vi "SelectWindow(SubVI).vi"(11 "Permanent data":T1) -> (0 "Error Out":errorcluster, 3 "Manometr out":T1)   [LabVIEW 2018]
uses:
  PressureGaugeInfo.ctl
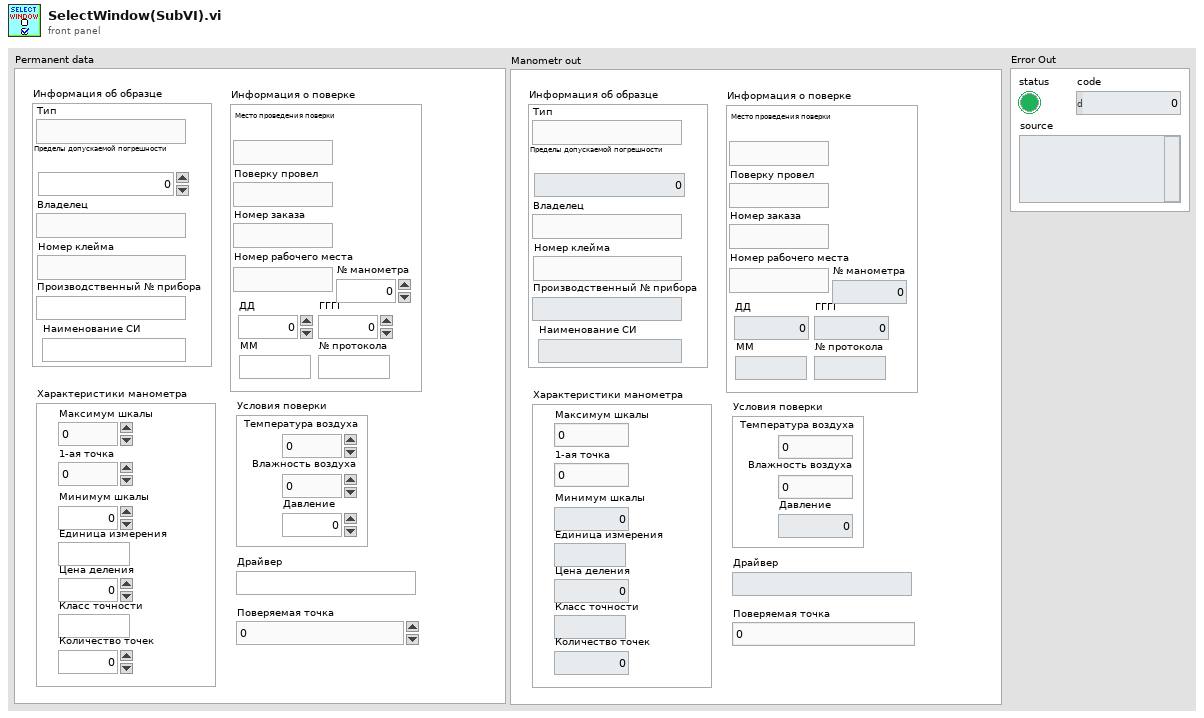
[diagram p1: front panel]
types:
  T1 = typedef "PressureGaugeInfo.ctl" = cluster{"Информация об образце":cluster{"Тип":string, "Владелец":string, "Номер клейма":string, "Пределы допускаемой погрешности ":dbl, "Производственный № прибора":string, "Наименование СИ":string}, "Информация о поверке":cluster{"Место проведения поверки":string, "Поверку провел":string, "Номер заказа":string, "Номер рабочего места":string, "ДД":dbl, "ММ":string, "ГГГГ":dbl, "№ протокола":string, "№ манометра":dbl}, "Характеристики манометра":cluster{"Максимум шкалы":dbl, "1-ая точка":dbl, "Единица измерения":string, "Цена деления":dbl, "Класс точности":string, "Минимум шкалы":dbl, "Количество точек":dbl}, "Условия поверки":cluster{"Температура воздуха":dbl, "Влажность воздуха":dbl, "Давление":dbl}, "Драйвер":string, "Поверяемая точка":dbl}
  T2 = typedef "LVRectTypeDef.ctl" = cluster{"Left":i16, "Top":i16, "Right":i16, "Bottom":i16}
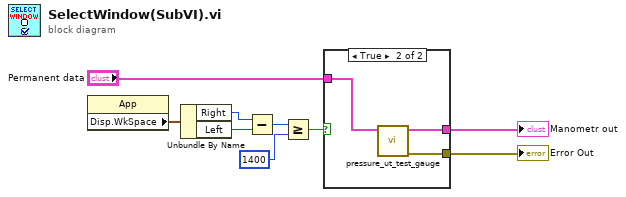
[diagram p0: block diagram]
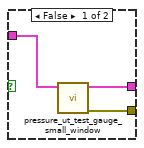
[diagram p2: hidden frame]
diagram:
  n1 = property class="App"() -> ("Disp.WkSpace"=w9:T2)  [unwired: 2 in, 2 out]
  n2 = Unbundle By Name(w9) -> ("Right"=w8:i16, "Left"=w7:i16)
  n3 = Subtract(x=w8, y=w7) -> (x-y=w6:i16)
  n4 = Greater Or Equal?(x=w6, y=i16 1400) -> (x >= y?=w4:bool)
  n5 = case shown="True" w4 {
    tunnel: "Permanent data" -> [w12 w15]
    tunnel: [w11 w14] -> w2
    tunnel: [w10 w13] -> w1
    frame False {
      n6 = call "pressure_ut_test_gauge_small_window.vi"("Manometr in"=w12) -> ("Error Out"=w10:errorcluster, "Manometr out"=w11:T1)  [unwired: 9 in]
    }
    frame True {
      n7 = call "pressure_ut_test_gauge.vi"("Manometr in"=w15) -> ("Error Out"=w13:errorcluster, "Manometr out"=w14:T1)  [unwired: 9 in]
    }
  }
  "Manometr out" <- w2
  "Error Out" <- w1
